vi "Get Camera Event Status.vi"(8 "error in (no error)":errorcluster, 11 "camStatus":u32) -> (0 "error out":errorcluster, 2 "function return":u32, 3 "camStatus out":u32)   [LabVIEW 2014, in "atmcd32d.lvlib"]
doc: "unsigned int WINAPI GetCameraEventStatus(DWORD * camStatus);"
uses:
  atmcd32d.lvlib
  atmcd32d.dll
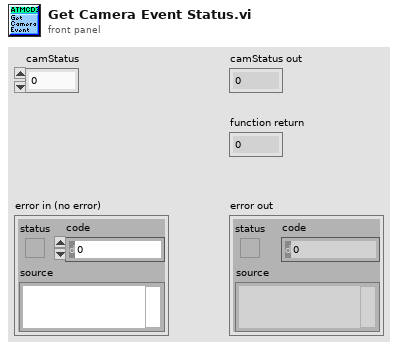
[diagram p1: front panel]
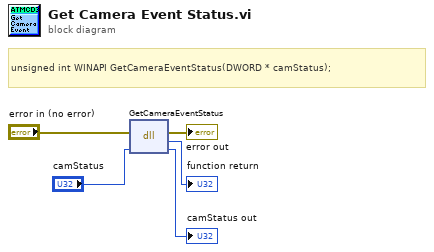
[diagram p0: block diagram]
diagram:
  # "unsigned int WINAPI GetCameraEventStatus(DWORD * camStatus);"
  n1 = dll-call lib="C:/Users/Bakir/Documents/Lambda2-Testing/lib/Andorlib/atmcd32d.*" fn="GetCameraEventStatus"(error in="error in (no error)", "camStatus"="camStatus") -> (error out=→"error out":errorcluster, →"function return":u32, "camStatus"=→"camStatus out":u32)  [unwired: 2 in, 1 out]
